vi "BRig_Host_comm_TCP_testConnect.vi"() -> ()   [LabVIEW 2014]
panel:
  out "error out":errorcluster
  in  "stop":bool
  out "Connected":bool
  out "Listening":bool
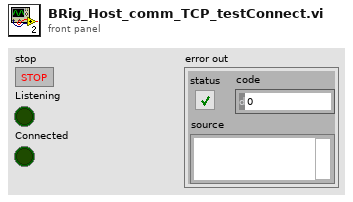
[diagram p1: front panel]
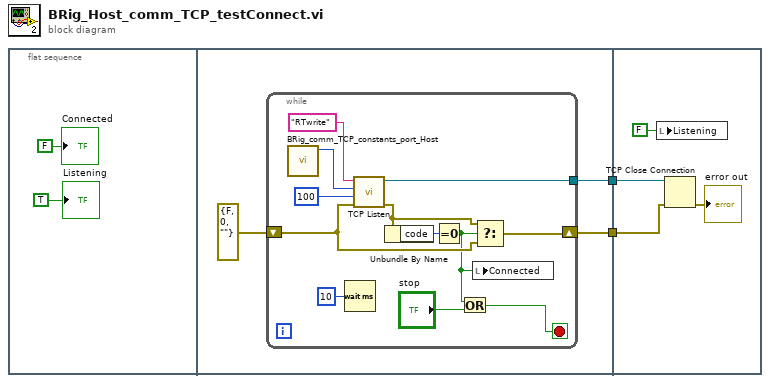
[diagram p0: block diagram]
diagram:
  n1 = flat-sequence {
    tunnel: [w6] -> w2
    tunnel: [w5] -> w1
    tunnel: w2 -> [w22]
    tunnel: w1 -> [w21]
    frame #0 {
      "Listening" <- TRUE ("Listening")
      "Connected" <- FALSE ("Connected")
    }
    frame #1 {
      n2 = while {
        shift-right: [w13] -> w5
        shift-left: errorcluster {"status"=FALSE, "code"=0, "source"=""} ("error in (no error)") -> [w15]
        tunnel: [w12] -> w6
        stop <- w8 stop-if-true
        n3 = call "BRig_comm_TCP_constants_port_Host.vi"() -> ("output_TCP_port"=w19:u16)  [unwired: 11 in]
        n4 = Wait (ms)(milliseconds to wait=u32 10) -> ()  [unwired: 1 out]
        n5 = call <vilib>:"TCP Listen.vi"("error in (no error)"=w15, "timeout ms (wait forever: -1)"=100, "port"=w19, "service name"="RTwrite") -> ("error out"=w14:errorcluster, "connection ID"=w12:refnum<k5>)  [unwired: 3 in, 3 out]
        n6 = Unbundle By Name(w14) -> ("code"=w16:i32)
        n7 = Equal To 0?(x=w16) -> (x = 0?=w9:bool)
        n8 = Or(x=w9, y="stop") -> (x .or. y?=w8:bool)
        n9 = local write "Connected"(w9) -> ()
        n10 = Select(t=w14, s=w9, f=w15) -> (s? t:f=w13:errorcluster)
      }
    }
    frame #2 {
      n11 = local write "Listening"(FALSE ("Listening")) -> ()
      n12 = TCP Close Connection(connection ID=w22, error in (no error)=w21) -> (error out=→"error out":errorcluster)  [unwired: 1 in, 1 out]
    }
  }
